vi "lp-client.vi"() -> ()   [LabVIEW 2010]
uses:
  socket_type.ctl
  zmq_context.lvclass
  zmq_socket.lvclass
  zeromq.lvlib
panel:
  out "attempt":i32
  out "loop":string
  in  "stop":bool
  in  "ntries":i32=20
  out "reply":string[](array[string])
  in  "timeout":u32=100
  in  "endpoint":string="tcp://127.0.0.1:5555"
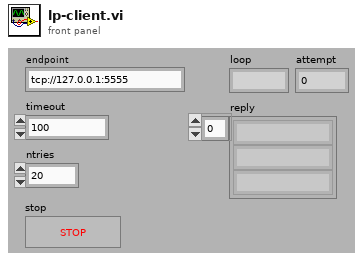
[diagram p1: front panel]
types:
  T1 = typedef "zeromq.lvlib/socket_type.ctl" = enum8{"ZMQ_PAIR", "ZMQ_PUB", "ZMQ_SUB", "ZMQ_REQ", "ZMQ_REP", "ZMQ_DEALER", "ZMQ_ROUTER", "ZMQ_PULL", "ZMQ_PUSH", "ZMQ_XPUB", "ZMQ_XSUB"}
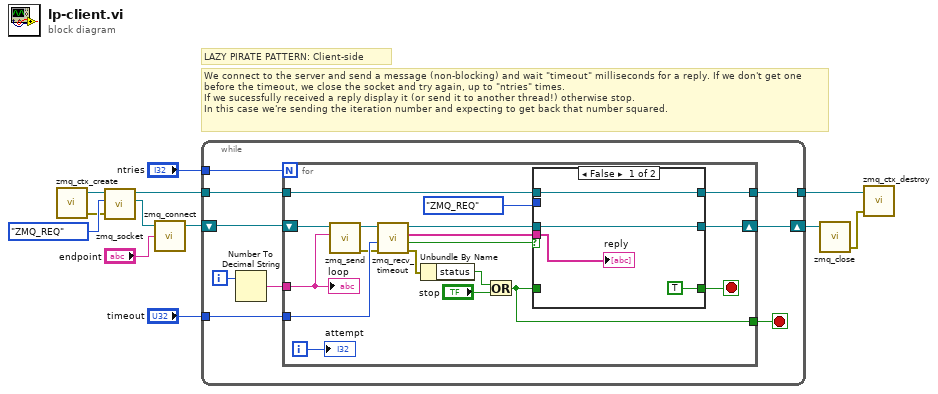
[diagram p0: block diagram]
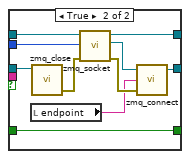
[diagram p2: hidden frame]
diagram:
  # "We connect to the server and send a message (non-blocking) and wait \"timeout\" milliseconds for a reply. If we don't get one before the timeout, we close the socket and try again, up to \"ntries\" times.\nIf we sucessfully received a reply display it (or send it to another thread!) otherwise stop.\nIn this case we're sending the iteration number and expecting to get back that number squared."
  # "LAZY PIRATE PATTERN: Client-side"
  n1 = call "zmq_ctx_create.vi"() -> ("error out"=w1:errorcluster, "context out"=w10:refnum<class "zmq_context.lvclass">)  [unwired: 4 in]
  n2 = call "zmq_socket.vi"("error in"=w1, "socket type"=socket_type."ZMQ_REQ", "context in"=w10) -> ("socket out"=w8:refnum<class "zmq_socket.lvclass">, "context out"=w7:refnum<class "zmq_context.lvclass">)  [unwired: 2 in, 1 out]
  n3 = call "zmq_connect.vi"("endpoint"="endpoint", "socket in"=w8) -> ("socket out"=w5:refnum<class "zmq_socket.lvclass">)  [unwired: 2 in, 1 out]
  n4 = while {
    tunnel: w7 -> [w21]
    tunnel: "timeout" -> [w20]
    tunnel: "ntries" -> [w19]
    tunnel: [w14] -> w4
    shift-right: [w13] -> w3
    shift-left: w5 -> [w15]
    i -> [w18]
    stop <- w16 stop-if-true
    n5 = Number To Decimal String(number=w18) -> (decimal integer string=w17:string)  [unwired: 1 in]
    n6 = for {
      N: w19 -> [_]
      tunnel: w21 -> [w25]
      tunnel: w20 -> [w38]
      tunnel: w17 -> [w34]
      tunnel: [w28] -> w16
      shift-right: [w24] -> w13
      shift-left: w15 -> [w26]
      tunnel: [w23] -> w14
      i -> [w33]
      stop <- w27 stop-if-true
      n7 = call "zmq_send.vi"("data"=w34, "socket in"=w26) -> ("error out"=w35:errorcluster, "socket out"=w36:refnum<class "zmq_socket.lvclass">)  [unwired: 5 in]
      n8 = call "zmq_recv_timeout.vi"("error in"=w35, "timeout (ms)"=w38, "socket in"=w36) -> ("error out"=w32:errorcluster, "timeout?"=w31:bool, "parts"=w37:string[], "socket out"=w39:refnum<class "zmq_socket.lvclass">)  [unwired: 1 in]
      n9 = Unbundle By Name(w32) -> ("status"=w30:bool)
      n10 = Or(x=w30, y="stop") -> (x .or. y?=w28:bool)
      n11 = case shown="False" w31 {
        tunnel: w39 -> [w41 w53]
        tunnel: w37 -> [w43 _]
        tunnel: w28 -> [_ w52]
        tunnel: [TRUE w52] -> w27
        tunnel: w25 -> [w40 w51]
        tunnel: [w41 w46] -> w24
        tunnel: [w40 w48] -> w23
        tunnel: socket_type."ZMQ_REQ" ("socket type") -> [_ w45]
        frame False {
          "reply" <- w43
        }
        frame True {
          n12 = local read "endpoint"() -> (w44:string)
          n13 = call "zmq_close.vi"("socket"=w53) -> ("error out"=w50:errorcluster)  [unwired: 4 in]
          n14 = call "zmq_socket.vi"("error in"=w50, "socket type"=w45, "context in"=w51) -> ("error out"=w49:errorcluster, "socket out"=w47:refnum<class "zmq_socket.lvclass">, "context out"=w48:refnum<class "zmq_context.lvclass">)  [unwired: 2 in]
          n15 = call "zmq_connect.vi"("error in"=w49, "endpoint"=w44, "socket in"=w47) -> ("socket out"=w46:refnum<class "zmq_socket.lvclass">)  [unwired: 1 in, 1 out]
        }
      }
      "loop" <- w34
      "attempt" <- w33
    }
  }
  n16 = call "zmq_close.vi"("socket"=w3) -> ("error out"=w2:errorcluster)  [unwired: 4 in]
  n17 = call "zmq_ctx_destroy.vi"("error in"=w2, "context in"=w4) -> ()  [unwired: 3 in, 1 out]
